vi "Init.vi"(8 "Implemented Msgs":T1, 9 "Is Normal":bool, 10 "Self":refnum<user-event>) -> (3 "Created Info out":refnum<class "Created Info.lvclass">)   [LabVIEW 2021, in "jettl.lvlib" / "Actor.lvlib" / "Created Info.lvclass"]
uses:
  Created Info.lvclass
  Msg/Msg.lvclass
  Utilities/Implemented Msgs.ctl
  Created Info.lvclass/Created Info.ctl
  Utilities/Utilities.lvlib
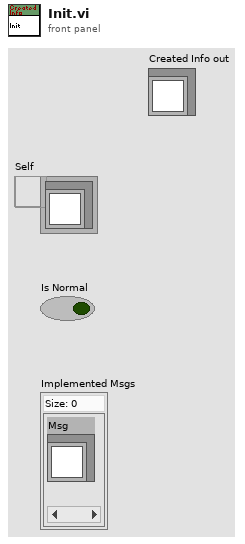
[diagram p1: front panel]
types:
  T1 = typedef "jettl.lvlib/Utilities.lvlib/Implemented Msgs.ctl" = set{refnum<class "Msg.lvclass">}
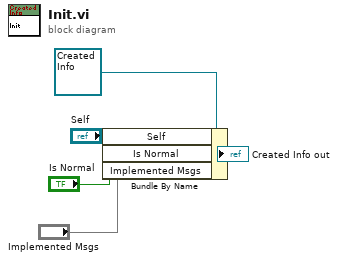
[diagram p0: block diagram]
diagram:
  n1 = Bundle By Name(cluster=refnum<class "Created Info.lvclass"> refnum ("Created Info out"), "Self"="Self", "Is Normal"="Is Normal", "Implemented Msgs"="Implemented Msgs") -> (→"Created Info out":refnum<class "Created Info.lvclass">)
